vi "Read.vi"(11 "ApiValue in":refnum<class "ApiValue.lvclass">) -> (2 "API":refnum<class "API.lvclass">)   [LabVIEW 2020, in "Volatus.lvlib" / "ApiValue.lvclass"]
uses:
  ApiValue.lvclass
  ApiValue.lvclass/ApiValue.ctl
  API/API.lvclass
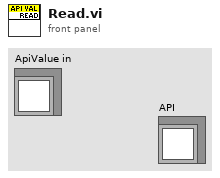
[diagram p1: front panel]
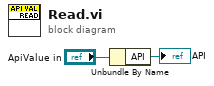
[diagram p0: block diagram]
diagram:
  n1 = Unbundle By Name("ApiValue in") -> ("API"=→"API":refnum<class "API.lvclass">)
